vi "ReinitializeCtls.vi"(8 "error in (no error)":errorcluster, 10 "Control Array In":string[](array[string]), 11 "CtlLookup In":T1) -> (0 "error in (no error) Out":errorcluster, 3 "CtlLookup Out":T1)   [LabVIEW 2018, in "CtlReferences.lvlib" / "CtlReferences.lvclass"]
doc: "Reinitialized specified control names to default values"
uses:
  CtlReferences.lvclass
  TypeDefs/CtlLookup.ctl
  CtlReferences.lvclass/CtlReferences.ctl
  GetControlRef/GetControl_Control.vi
  GetControlRef/GetCtlRef_Base.vi
  GetCtlRef_Lookup.vi
  <vilib>/Utility/error.llb/Error Cluster From Error Code.vi
  Error_ToSpecificClass.vi
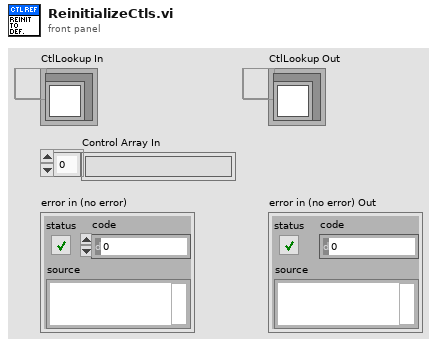
[diagram p1: front panel]
types:
  T1 = typedef "CtlReferences.lvlib/CtlReferences.lvclass/CtlLookup.ctl" = refnum<data-value>
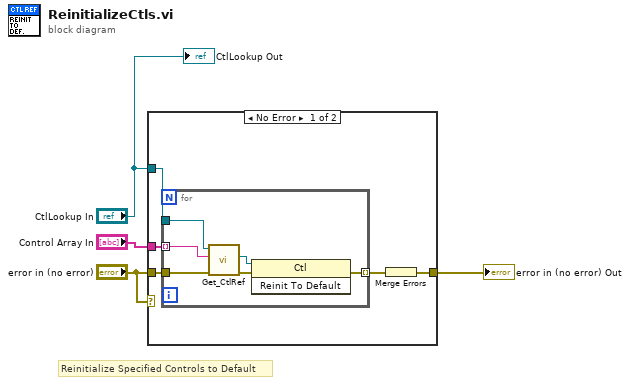
[diagram p0: block diagram]
diagram:
  # "Reinitialize Specified Controls to Default"
  n1 = case shown="No Error" "error in (no error)" {
    tunnel: "error in (no error)" -> [w9 w16]
    tunnel: [w7 w16] -> w4
    tunnel: "Control Array In" -> [w6 _]
    tunnel: "CtlLookup In" -> [w5 _]
    frame No Error {
      n2 = for {
        tunnel: w9 -> [w15]
        tunnel: w6 -> [w14] mode=indexing
        tunnel: w5 -> [w13]
        tunnel: [w10] -> w8 mode=indexing
        n3 = call-poly "Get_CtlRef.vi"("error in (no error)"=w15, "Control Label"=w14, "CtlLookup In"=w13) -> ("error out"=w11:errorcluster, "Reference Out"=w12:refnum<vi>)  [unwired: 6 in, 1 out]
        n4 = invoke class="Ctl" method="Reinit To Default"(reference=w12, error in=w11) -> (error out=w10:errorcluster)  [unwired: 1 in, 2 out]
      }
      n5 = Merge Errors(w8) -> (w7:errorcluster)
    }
    frame Error {
    }
  }
  "error in (no error) Out" <- w4
  "CtlLookup Out" <- "CtlLookup In"
